vi "Test Returns Default.vi"() -> ()   [LabVIEW 2017]
uses:
  77b9375a-903b-4822-a833-e4a9df312311.vi
  JSON text to Variant.vi
  <vilib>/addons/_JKI Toolkits/Caraya/classes/Test/Test.lvclass
  <vilib>/addons/_JKI Toolkits/Caraya/classes/Assert/Assert.lvclass
panel:
  out "Array 2":errorcluster[](array[cluster])
  out "Array":cluster{"A":i32, "sub":cluster{"A":i32}}[](array[cluster])
  out "Variant":variant
  out "Should be True":bool[](array[boolean])
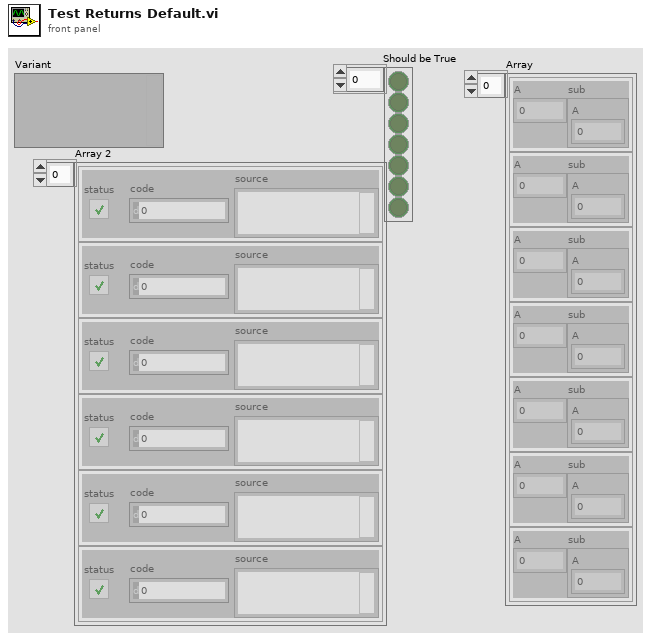
[diagram p1: front panel]
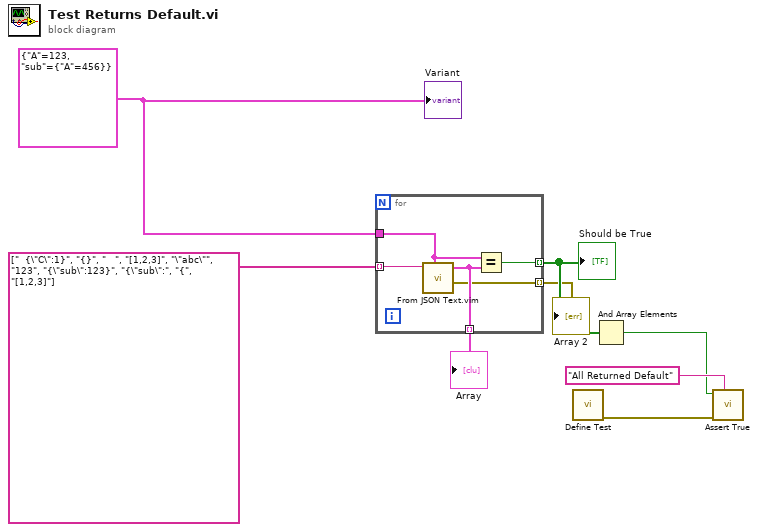
[diagram p0: block diagram]
diagram:
  w3 = cluster{"A":i32, "sub":cluster{"A":i32}} {"A"=123, "sub"={"A"=456}}
  n1 = for {
    tunnel: string[] ["  {\"C\":1}", "{}", "   ", "[1,2,3]", "\"abc\"", "123", "{\"sub\":123}", "{\"sub\":", "{", "[1,2,3]"] ("JSON") -> [w13] mode=indexing
    tunnel: w3 -> [w12]
    tunnel: [w11] -> w4 mode=indexing
    tunnel: [w10] -> w2 mode=indexing
    tunnel: [w9] -> w1 mode=indexing
    n2 = call "From JSON Text.vim"("Data Type and Default Value"=w12, "JSON"=w13) -> ("error out"=w9:errorcluster, "Data out"=w10:cluster{"A":i32, "sub":cluster{"A":i32}})  [unwired: 8 in]
    n3 = Equal?(x=w12, y=w10) -> (x = y?=w11:bool)
  }
  "Should be True" <- w4
  "Array" <- w2
  "Array 2" <- w1
  n4 = call <vilib>:"Define Test.vi"() -> ("error out"=w6:errorcluster)  [unwired: 11 in]
  n5 = And Array Elements(Boolean array=w4) -> (logical AND=w5:bool)
  n6 = call <vilib>:"Assert True.vi"("Label"="All Returned Default", "error in (no error)"=w6, "True?"=w5) -> ()  [unwired: 8 in, 1 out]
  "Variant" <- w3
